vi "Remove Key.vi"(7 "Section Name":string, 8 "error in (no error)":errorcluster, 10 "Key Name":string, 11 "Config in":refnum<class "LabVIEW-Config.lvclass">) -> (0 "error out":errorcluster, 2 "Key Found?":bool, 3 "Config out":refnum<class "LabVIEW-Config.lvclass">)   [LabVIEW 2017, in "LabVIEW-Config.lvlib" / "LabVIEW-Config.lvclass"]
uses:
  LabVIEW-Config.lvclass
  LabVIEW-Config.lvclass/LabVIEW-Config.ctl
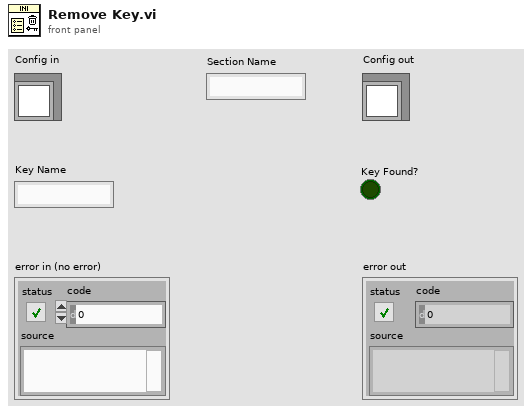
[diagram p1: front panel]
types:
  T1 = typedef "LabVIEW-Config.lvlib/LabVIEW-Config.lvclass/KeyInfo.ctl" = cluster{"Key Indexes":cluster{"Indexes":i32[]}[], "Session Found?":bool, "Key found?":bool, "Session Index":i32}
  T2 = typedef "LabVIEW-Config.lvlib/LabVIEW-Config.lvclass/LineToken.ctl" = enum8{"comment", "section", "key", "more"}
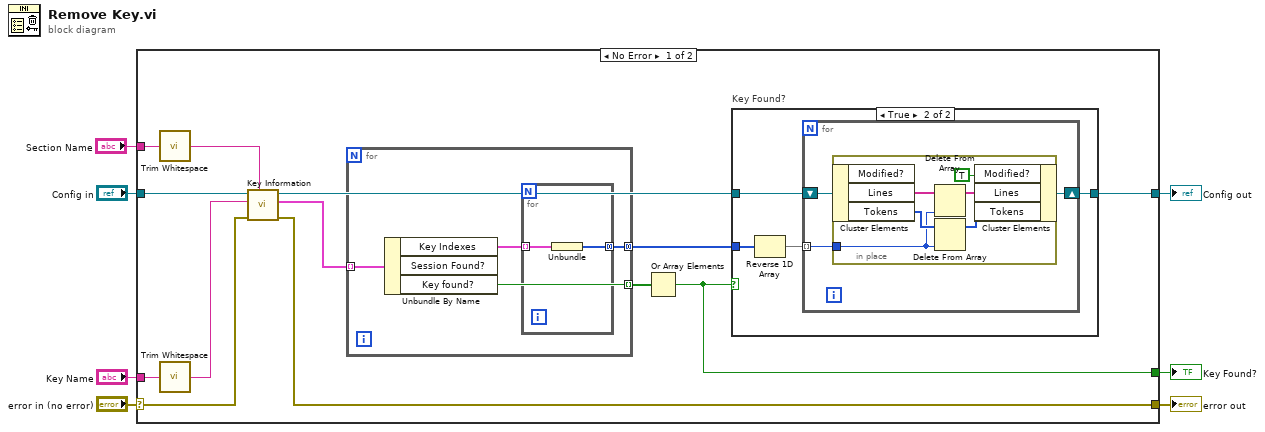
[diagram p0: block diagram]
diagram:
  n1 = case shown="No Error" "error in (no error)" {
    selector: "error in (no error)" -> [w15 w42]
    tunnel: "Config in" -> [w19 w41]
    tunnel: [w14 w42] -> w6
    tunnel: [w20 w41] -> w4
    tunnel: "Section Name" -> [w17 _]
    tunnel: [w8 _] -> w2
    tunnel: "Key Name" -> [w16 _]
    frame No Error {
      n2 = call <vilib>:"Trim Whitespace.vi"("string"=w17) -> ("trimmed string"=w9:string)  [unwired: 1 in]
      n3 = call <vilib>:"Trim Whitespace.vi"("string"=w16) -> ("trimmed string"=w10:string)  [unwired: 1 in]
      n4 = call "Key Information.vi"("Section Name"=w9, "error in (no error)"=w15, "Key Name"=w10, "Config in"=w19) -> ("error out"=w14:errorcluster, "Key Information"=w13:T1[], "Config out"=w18:refnum<class "LabVIEW-Config.lvclass">)  [unwired: 5 in]
      n5 = for {
        tunnel: w13 -> [w24] mode=indexing
        tunnel: [w23] -> w12 mode=indexing
        tunnel: [w21] -> w11 mode=concatenating
        n6 = Unbundle By Name(w24) -> ("Key Indexes"=w22:cluster{"Indexes":i32[]}[], "Key found?"=w23:bool)  [unwired: 1 out]
        n7 = for {
          tunnel: w22 -> [w26] mode=indexing
          tunnel: [w25] -> w21 mode=concatenating
          n8 = Unbundle(w26) -> ("Indexes"=w25:i32[])
        }
      }
      n9 = Or Array Elements(Boolean array=w12) -> (logical OR=w8:bool)
      n10 = case "Key Found?" shown="True" w8 {
        tunnel: [w27 w31] -> w20
        tunnel: w18 -> [w27 w30]
        tunnel: w11 -> [_ w29]
        frame False {
        }
        frame True {
          n11 = Reverse 1D Array(array=w29) -> (reversed array=w28:i32[])
          n12 = for {
            tunnel: w28 -> [w32] mode=indexing
            shift-right: [w34] -> w31
            shift-left: w30 -> [w33]
            n13 = in-place {
              in-place-border: w32 -> [w35]
              n14 = in-place-cluster #1(w33) -> ("Lines"=w39:string[], "Tokens"=w38:T2[])  [unwired: 1 out]
              n15 = Delete From Array(array=w39, index=w35) -> (array with subset deleted=w36:string[])  [unwired: 1 in, 1 out]
              n16 = Delete From Array(array=w38, index=w35) -> (array with subset deleted=w37:T2[])  [unwired: 1 in, 1 out]
              n17 = in-place-cluster #1("Modified?"=TRUE, "Lines"=w36, "Tokens"=w37) -> (w34:refnum<class "LabVIEW-Config.lvclass">)
            }
          }
        }
      }
    }
    frame Error {
    }
  }
  "error out" <- w6
  "Config out" <- w4
  "Key Found?" <- w2
